vi "Write.Buffer.vi"(8 "error in":errorcluster, 9 "Offset":i32, 10 "Values":dbl[](array[numeric]), 11 "Write in":refnum<class "Write.lvclass">) -> (0 "error out":errorcluster, 3 "Write out":refnum<class "Write.lvclass">)   [LabVIEW 2024, in "VS Plugin Data Access Engine.lvlib" / "Write.lvclass"]
uses:
  Write.lvclass
  Write.lvclass/Write.ctl
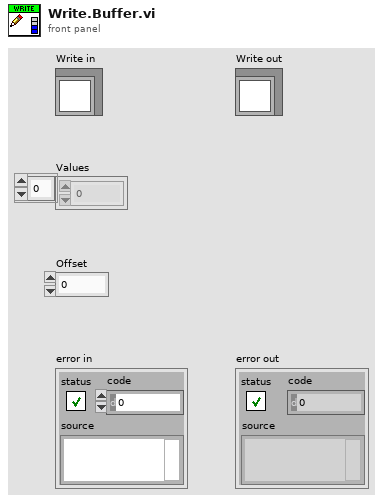
[diagram p1: front panel]
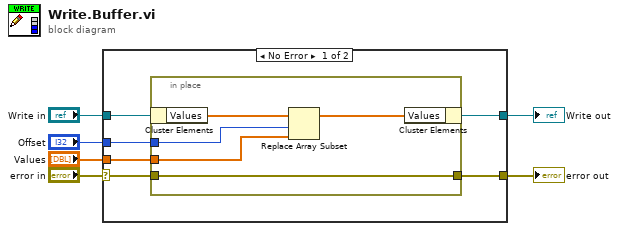
[diagram p0: block diagram]
diagram:
  n1 = case shown="No Error" "error in" {
    selector: "error in" -> [w12 w19]
    tunnel: [w11 w19] -> w5
    tunnel: [w9 w18] -> w1
    tunnel: "Write in" -> [w10 w18]
    tunnel: "Offset" -> [w8 _]
    tunnel: "Values" -> [w7 _]
    frame No Error {
      n2 = in-place {
        in-place-border: w7 -> [w16]
        in-place-border: w12 -> [w17]
        in-place-border: [w17] -> w11
        in-place-border: w8 -> [w13]
        n3 = in-place-cluster #1(w10) -> ("Values"=w15:dbl[])
        n4 = Replace Array Subset(array=w15, new element=w16, index=w13) -> (w14:dbl[])
        n5 = in-place-cluster #1("Values"=w14) -> (w9:refnum<class "Write.lvclass">)
      }
    }
    frame Error {
    }
  }
  "error out" <- w5
  "Write out" <- w1
